vi "NewExperimentDialog.vi"(8 "error in (no error)":errorcluster, 11 "File Path":path=path "E:/LINKAM Measurements_Naama") -> (0 "error out":errorcluster, 1 "Goal 2":string, 2 "File Path 2":path=path "E:/LINKAM Measurements_Naama/200514", 3 "Experiment Name 2":string="t", 4 "Add Entry Pressed?":bool=TRUE)   [LabVIEW 2013]
doc: "Use this template to build a VI to use as a subVI."
panel:
  in  "Get focus":string
  in  "Goal":string
  in  "Experiment Name":string
  in  "Cancel Button":bool
  in  "Add Entry Button":bool
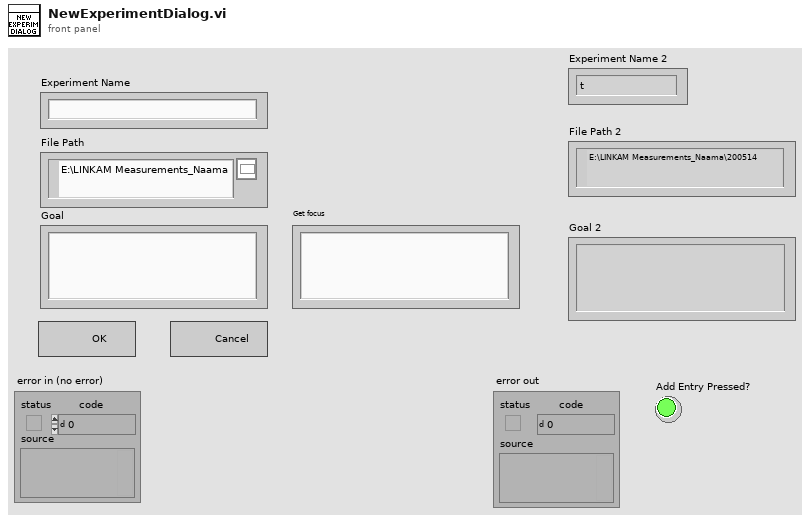
[diagram p1: front panel]
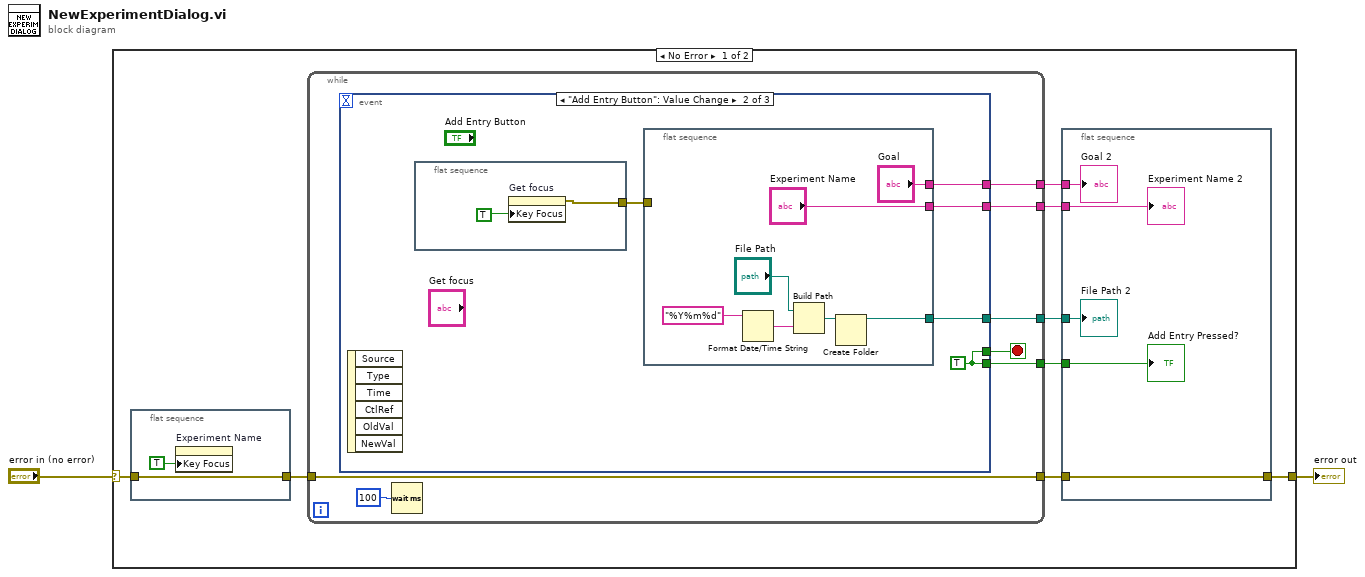
[diagram p0: block diagram]
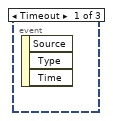
[diagram p2: hidden frame]
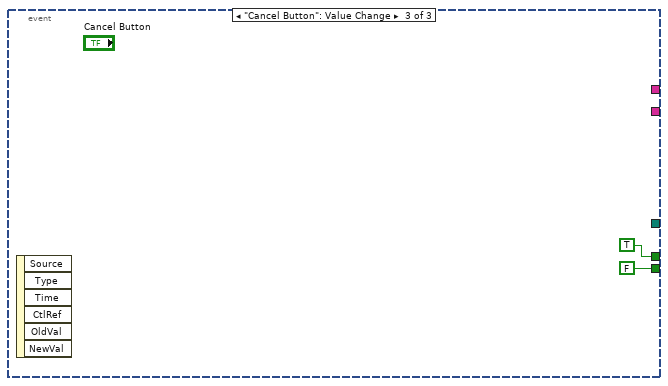
[diagram p3: hidden frame]
diagram:
  n1 = case shown="No Error" "error in (no error)" {
    selector: "error in (no error)" -> [w6 w41]
    tunnel: [w4 w41] -> w1
    frame No Error {
      n2 = flat-sequence {
        tunnel: w6 -> [w16]
        tunnel: [w16] -> w5
        frame #0 {
          n3 = property on="Experiment Name" class="Str"("Key Focus"=TRUE) -> ()  [unwired: 2 in, 2 out]
        }
      }
      n4 = while {
        tunnel: [w23] -> w10
        tunnel: [w21] -> w9
        tunnel: [w20] -> w8
        tunnel: [w19] -> w7
        tunnel: w5 -> [w18]
        tunnel: [w18] -> w3
        stop <- w24 stop-if-true
        n5 = event shown="[1] \"Add Entry Button\": Value Change" {
          selector: _ -> [_ _ _]
          dyn-events: _ -> [_ _ _]
          timeout: _ -> [_ _ _]
          tunnel: [_ w29 TRUE] -> w24
          tunnel: [_ w29 FALSE] -> w23
          tunnel: [_ w28 _] -> w21
          tunnel: [_ w26 _] -> w20
          tunnel: [_ w27 _] -> w19
          event Timeout {
            n6 = event-data() -> ()  [unwired: 1 in, 3 out]
          }
          event "Add Entry Button": Value Change {
            w29 = TRUE
            n7 = event-data() -> ()  [unwired: 1 in, 6 out]
            n8 = flat-sequence {
              tunnel: [w31] -> w25
              frame #0 {
                n9 = property on="Get focus" class="Str"("Key Focus"=TRUE) -> (error out=w31:errorcluster)  [unwired: 2 in, 1 out]
              }
            }
            n10 = flat-sequence {
              tunnel: ["Experiment Name"] -> w28
              tunnel: ["Goal"] -> w27
              tunnel: [w33] -> w26
              tunnel: w25 -> [_]
              frame #0 {
                n11 = Format Date/Time String(time format string (%c)="%Y%m%d") -> (date/time string=w35:string)  [unwired: 2 in]
                n12 = Build Path(base path="File Path", name or relative path=w35) -> (appended path=w32:path)
                n13 = Create Folder(path (use dialog)=w32) -> (created path=w33:path)  [unwired: 2 in, 2 out]
              }
            }
          }
          event "Cancel Button": Value Change {
            n14 = event-data() -> ()  [unwired: 1 in, 6 out]
          }
        }
        n15 = Wait (ms)(milliseconds to wait=u32 100) -> ()  [unwired: 1 out]
      }
      n16 = flat-sequence {
        tunnel: w10 -> [w15]
        tunnel: w9 -> [w14]
        tunnel: w8 -> [w13]
        tunnel: w7 -> [w12]
        tunnel: w3 -> [w11]
        tunnel: [w11] -> w4
        frame #0 {
          "Add Entry Pressed?" <- w15
          "Experiment Name 2" <- w14
          "File Path 2" <- w13
          "Goal 2" <- w12
        }
      }
    }
    frame Error {
    }
  }
  "error out" <- w1
